vi "Apply Gradients.vi"(10 "Hardware Parameters In":T2={"Scan Calibration [G/V]"=0.0, "Modulation Calibration [G/V]"=0.0, "Modulation Phase [deg]"=0.0, "Modulation Frequency [Hz]"=0.0, "Attenuation [dB]"=0, "Input Channel Count"=0, "Time constant"=7, "Sensitivity"=17, "Frequency Output Voltage [V]"=0.0, "Phase Output Voltage [V]"=0.0, "Lock-in Offset Compensation"=FALSE, "RF [GHz]"=0.0, "Q Start"=0.0, "Q End"=0.0, "Balance"=0.0, "Phase Error"=0.0, "AFC Error"=0.0, "AFC"=FALSE, "Magnet Rotation"=FALSE, "Balance Scaling Factor"=1.0, "Phase Error Scaling Factor"=1.0, "AFC Error Scaling Factor"=1.0, "Frequency Counter ID"="", "Sweep Waveform"=enum."Sawtooth", "Q-Factor Scale"=0.0, " Q-Data Scale"=0.0, " Q-Data Offset"=0.0, "Magnet Rotation Slope"=0.0, "Magnet Rotation Offset"=0.0, "Phase Sweep Resolution"=0.0, "Hardware Version Number"="", "Spectrometer ID Number"=0, "Spectrometer Name"="", "Lock in Saturation"=0.0, "Balance Threshold"=0.0, "Phase Error Threshold"=0.0, "AFC Error Threshold"=0.0, "Linear Actuator Length"=0.0, "Lock-in OK?"=FALSE, "Ignore Lock-in Comm. Failure"=FALSE, "Gradient Addresses"=[], "Gradient Calibrations [G/A*mm]"=[], "Gradient Power Supplies"=[], "Lock-in Address"="", "Magnet Type"=enum."RRI", "Camera Names"=[], "Sweep Limit [Gauss]"=0.0, "Modulation Limit [Gauss]"=0.0, "Balance Threshold Exceeded?"=FALSE, "Phase Threshold Exceeded?"=FALSE, "AFC Threshold Exceeded?"=FALSE, "Consecutive Re-tune attempts"=0, "Reverse Sweep Slope [sec]"=0.0, "Reverse Sweep Offset [G]"=0.0, "AFC Field Correction [V/MHz]"=0.0, "Active Gradients (X Y Z)"=[], "SpO2 Calibration [SpO2/V]"=1.0, "Heart Rate Calibration [BPM/V]"=1.0, "Thermocouple Channel"=""} {"Sensitivity" items=["", "2 nV", "5 nV", "10 nV", "20 nV", "50 nV", "100 nV", "200 nV", "500 nV", "1 uV", "2 uV", "5 uV", "10 uV", "20 uV", "50 uV", "100 uV", "200 uV", "500 uV", "1 mV", "2 mV", "5 mV", "10 mV", "20 mV", "50 mV", "100 mV", "200 mV", "500 mV", "1 V"]; "Time constant" items=["10 us", "20 us", "40 us", "80 us", "160 us", "320 us", "640 us", "5 ms", "10 ms", "20 ms", "50 ms", "100 ms", "200 ms", "500 ms", "1 s", "2 s", "5 s", "10 s", "20 s", "50 s", "100 s", "200 s", "500 s", "1 ks", "2 ks", "5 ks", "10 ks", "20 ks", "50 ks", "100 ks"]}, 11 "Acquisition Parameters In":T1={"Magnet Angle [deg]"=0.0, "Magnet Angles [deg]"=[], "DeltaVpp [v]"=0.0, "SEM [v]"=0.0, "DeltaVpp Thresh [v]"=0.0, "SEM Thresh [v]"=0.0, "Adaptive Processing"=FALSE, "Acquire Q"=FALSE, "Acquire Photos"=FALSE, "Adaptive Tuning"=FALSE, "Automated Matching"=FALSE, "X-Gradient [G/mm]"=0.0, "Y-Gradient [G/mm]"=0.0, "Z-Gradient [G/mm]"=0.0, "Central Field [G]"=0.0, "Scan Width [G]"=0.0, "Mod. Amp. [G]"=0.0, "Scan Time [s]"=0.0, "Pre-Scan Delay [ms]"=0, "Measurement Timeout [s]"=0.0, "Electromagnet Main Field [G]"=0.0, "Locked Central Field [G]"=0.0, "Scans Excluded"=0, "Scans Completed"=0, "No. Scans/Set"=0, "No. Scans for SNR"=0, "Field Locked Frequency [GHz]"=0.0, "Auto Set-based Field Center"=FALSE, "Prompt for oxy acquisition updates"=FALSE, "Oxy QA Scan?"=FALSE, "Exclude Bad Data"=FALSE, "Optimizing RF Power"=FALSE, "Gradients on/off"=FALSE, "Running Script"=TRUE, "Opto-Coupler Current [A]"=0.0, "Continuous Sweeping"=FALSE, "Sweep Rise Time [sec]"=0, "Reverse Sweep Central Field [G]"=0.0, "Forward Sweep Central Field [G]"=0.0, "Sweep Calibrated"=FALSE, "Modulation Calibrated"=FALSE, "First CheckCal Scan?"=FALSE, "AFC Field Correction"=FALSE, "OxyQAInit Scan Width [G]"=0.0, "OxyQAInit Mod. Amp. [G]"=0.0, "Scans Completed/Session"=0, "Acquire SpO2"=FALSE, "Acquire Temperature"=FALSE, "Over Mod"=FALSE} {"OxyQAInit Mod. Amp. [G]" min=0.0; "OxyQAInit Scan Width [G]" min=0.0; "Mod. Amp. [G]" min=0.0; "Scan Width [G]" min=0.0; "Measurement Timeout [s]" min=0.0; "Scan Time [s]" min=0.0; "Z-Gradient [G/mm]" min=0.0; "Y-Gradient [G/mm]" min=0.0; "X-Gradient [G/mm]" min=0.0; "SEM Thresh [v]" min=0.0; "DeltaVpp Thresh [v]" min=0.0; "SEM [v]" min=0.0}) -> (0 "error out":errorcluster)   [LabVIEW 2016]
uses:
  Types/Hardware Parameters.ctl
  Types/Acquisition Parameters.ctl
panel:
  # "Gradients"
  # "Field"
  # "Scans and Sets"
  # "Timing"
  # "Adaptive Dosimetric \nData Processing"
  # "Bridge I/O"
  # "Magnet Rotation"
  # "Field Calibration"
  # "Lock In Amplifier"
  # "Spectrometer Information"
  # "DAQ Settings"
  # "Gradient Coils and Field"
  # "X"
  # "Y"
  # "Z"
  # "Q-Measurements"
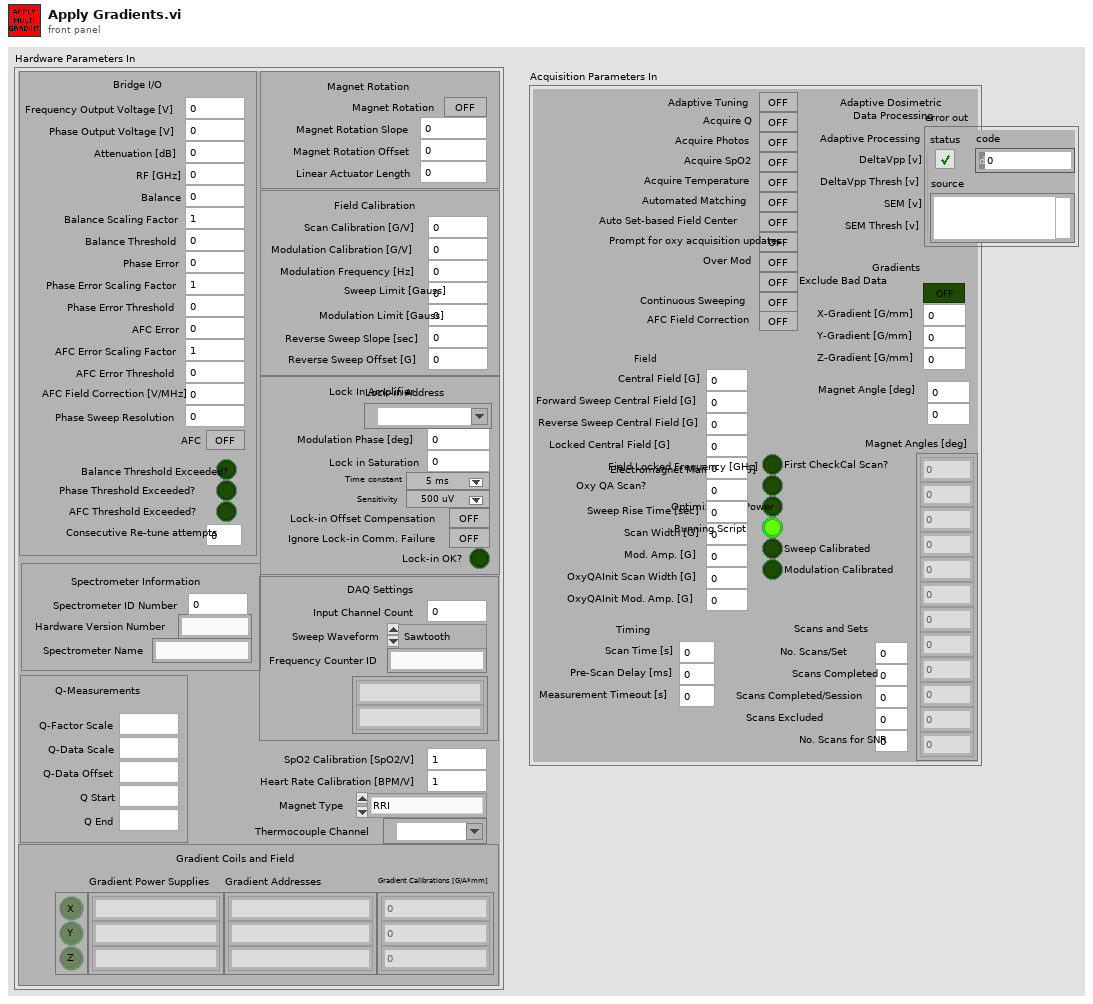
[diagram p1: front panel]
types:
  T1 = typedef "Acquisition Parameters.ctl" = cluster{"Magnet Angle [deg]":dbl, "Magnet Angles [deg]":dbl[], "DeltaVpp [v]":dbl, "SEM [v]":dbl, "DeltaVpp Thresh [v]":dbl, "SEM Thresh [v]":dbl, "Adaptive Processing":bool, "Acquire Q":bool, "Acquire Photos":bool, "Adaptive Tuning":bool, "Automated Matching":bool, "X-Gradient [G/mm]":dbl, "Y-Gradient [G/mm]":dbl, "Z-Gradient [G/mm]":dbl, "Central Field [G]":dbl, "Scan Width [G]":dbl, "Mod. Amp. [G]":dbl, "Scan Time [s]":dbl, "Pre-Scan Delay [ms]":u32, "Measurement Timeout [s]":dbl, "Electromagnet Main Field [G]":dbl, "Locked Central Field [G]":dbl, "Scans Excluded":u32, "Scans Completed":u32, "No. Scans/Set":u32, "No. Scans for SNR":u32, "Field Locked Frequency [GHz]":dbl, "Auto Set-based Field Center":bool, "Prompt for oxy acquisition updates":bool, "Oxy QA Scan?":bool, "Exclude Bad Data":bool, "Optimizing RF Power":bool, "Gradients on/off":bool, "Running Script":bool, "Opto-Coupler Current [A]":dbl, "Continuous Sweeping":bool, "Sweep Rise Time [sec]":u32, "Reverse Sweep Central Field [G]":dbl, "Forward Sweep Central Field [G]":dbl, "Sweep Calibrated":bool, "Modulation Calibrated":bool, "First CheckCal Scan?":bool, "AFC Field Correction":bool, "OxyQAInit Scan Width [G]":dbl, "OxyQAInit Mod. Amp. [G]":dbl, "Scans Completed/Session":u32, "Acquire SpO2":bool, "Acquire Temperature":bool, "Over Mod":bool}
  T2 = typedef "Hardware Parameters.ctl" = cluster{"Scan Calibration [G/V]":dbl, "Modulation Calibration [G/V]":dbl, "Modulation Phase [deg]":dbl, "Modulation Frequency [Hz]":dbl, "Attenuation [dB]":u16, "Input Channel Count":i32, "Time constant":u16, "Sensitivity":u16, "Frequency Output Voltage [V]":dbl, "Phase Output Voltage [V]":dbl, "Lock-in Offset Compensation":bool, "RF [GHz]":dbl, "Q Start":dbl, "Q End":dbl, "Balance":dbl, "Phase Error":dbl, "AFC Error":dbl, "AFC":bool, "Magnet Rotation":bool, "Balance Scaling Factor":dbl, "Phase Error Scaling Factor":dbl, "AFC Error Scaling Factor":dbl, "Frequency Counter ID":string, "Sweep Waveform":enum16{"Sine Wave", "Square Wave", "Sawtooth", "Triangle Wave"}, "Q-Factor Scale":dbl, " Q-Data Scale":dbl, " Q-Data Offset":dbl, "Magnet Rotation Slope":dbl, "Magnet Rotation Offset":dbl, "Phase Sweep Resolution":dbl, "Hardware Version Number":string, "Spectrometer ID Number":i32, "Spectrometer Name":string, "Lock in Saturation":dbl, "Balance Threshold":dbl, "Phase Error Threshold":dbl, "AFC Error Threshold":dbl, "Linear Actuator Length":dbl, "Lock-in OK?":bool, "Ignore Lock-in Comm. Failure":bool, "Gradient Addresses":string[], "Gradient Calibrations [G/A*mm]":dbl[], "Gradient Power Supplies":string[], "Lock-in Address":refnum<visa-resource-name>, "Magnet Type":enum16{"RRI", "BARDA", "Whole Body Permanent", "RRI Electromagnet"}, "Camera Names":string[], "Sweep Limit [Gauss]":dbl, "Modulation Limit [Gauss]":dbl, "Balance Threshold Exceeded?":bool, "Phase Threshold Exceeded?":bool, "AFC Threshold Exceeded?":bool, "Consecutive Re-tune attempts":i32, "Reverse Sweep Slope [sec]":dbl, "Reverse Sweep Offset [G]":dbl, "AFC Field Correction [V/MHz]":dbl, "Active Gradients (X Y Z)":bool[], "SpO2 Calibration [SpO2/V]":dbl, "Heart Rate Calibration [BPM/V]":dbl, "Thermocouple Channel":tag}
  T3 = enum16{"RRI", "BARDA", "Whole Body Permanent", "RRI Electromagnet"}
  T4 = enum16{"Main and Gradients", "Main Field", "Gradients"}
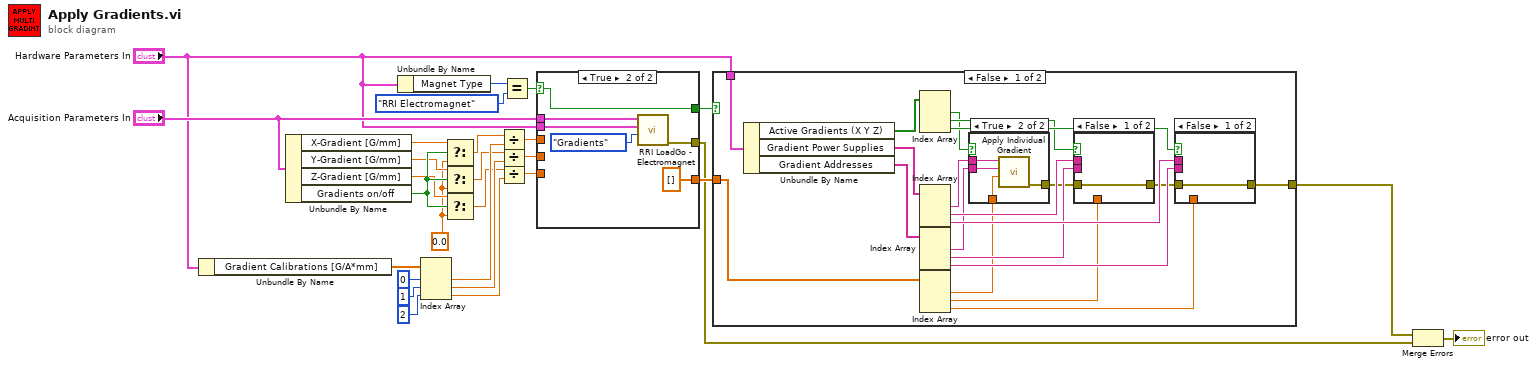
[diagram p0: block diagram]
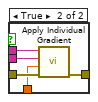
[diagram p2: hidden frame]
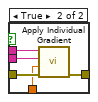
[diagram p3: hidden frame]
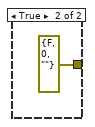
[diagram p5: hidden frame]
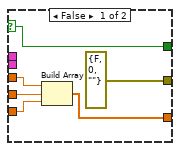
[diagram p6: hidden frame]
diagram:
  w1 = 0.0 ("t")
  n1 = Unbundle By Name("Hardware Parameters In") -> ("Gradient Calibrations [G/A*mm]"=w22:dbl[])
  n2 = Unbundle By Name("Acquisition Parameters In") -> ("X-Gradient [G/mm]"=w4:dbl, "Y-Gradient [G/mm]"=w3:dbl, "Z-Gradient [G/mm]"=w2:dbl, "Gradients on/off"=w8:bool)
  n3 = Unbundle By Name("Hardware Parameters In") -> ("Magnet Type"=w28:T3)
  n4 = Index Array(array=w22, index #1=0 ("index"), index #2=1 ("index"), index #3=2 ("index")) -> (element #1=w18:dbl, element #2=w17:dbl, element #3=w16:dbl)
  n5 = Select(t=w4, s=w8, f=w1) -> (s? t:f=w7:dbl)
  n6 = Select(t=w3, s=w8, f=w1) -> (s? t:f=w6:dbl)
  n7 = Select(t=w2, s=w8, f=w1) -> (s? t:f=w5:dbl)
  n8 = Divide(x=w7, y=w18) -> (x/y=w15:dbl)
  n9 = Divide(x=w6, y=w17) -> (x/y=w14:dbl)
  n10 = Divide(x=w5, y=w16) -> (x/y=w13:dbl)
  n11 = Equal?(x=w28, y=T3."RRI Electromagnet" ("Magnet Type")) -> (x = y?=w26:bool)
  n12 = case shown="True" w26 {
    selector: w26 -> [w33 w37]
    tunnel: "Acquisition Parameters In" -> [_ w35]
    tunnel: "Hardware Parameters In" -> [_ w39]
    tunnel: [errorcluster {"status"=FALSE, "code"=0, "source"=""} ("error out") w38] -> w10
    tunnel: [w33 w37] -> w25
    tunnel: w15 -> [w32 _]
    tunnel: w14 -> [w31 _]
    tunnel: w13 -> [w30 _]
    tunnel: [w29 dbl[] []] -> w12
    frame False {
      n13 = Build Array(w32, w31, w30) -> (w29:dbl[])
    }
    frame True {
      n14 = call "RRI LoadGo - Electromagnet.vi"("Control Coils"=T4."Gradients", "Hardware Parameters"=w39, "Acquisition Parameters"=w35) -> ("error out"=w38:errorcluster)  [unwired: 4 in]
    }
  }
  n15 = case shown="False" w25 {
    tunnel: [w48 errorcluster {"status"=FALSE, "code"=0, "source"=""} ("error out")] -> w11
    tunnel: "Hardware Parameters In" -> [w60 _]
    tunnel: w12 -> [w44 _]
    frame False {
      n16 = Unbundle By Name(w60) -> ("Active Gradients (X Y Z)"=w47:bool[], "Gradient Power Supplies"=w46:string[], "Gradient Addresses"=w45:string[])
      n17 = Index Array(array=w47) -> (element #1=w49:bool, element #2=w54:bool, element #3=w55:bool)  [unwired: 3 in]
      n18 = Index Array(array=w46) -> (element #1=w50:string, element #2=w58:string, element #3=w59:string)  [unwired: 3 in]
      n19 = Index Array(array=w45) -> (element #1=w51:string, element #2=w56:string, element #3=w57:string)  [unwired: 3 in]
      n20 = Index Array(array=w44) -> (element #1=w43:dbl, element #2=w42:dbl, element #3=w41:dbl)  [unwired: 3 in]
      n21 = case shown="True" w49 {
        tunnel: w50 -> [_ w76]
        tunnel: w51 -> [_ w75]
        tunnel: [_ w74] -> w52
        tunnel: w43 -> [_ w73]
        frame False {
        }
        frame True {
          n22 = call "Apply Individual Gradient.vi"("Current [A]"=w73, "Gradient Supply Address"=w75, "Gradient Supply Type"=w76) -> ("error out"=w74:errorcluster)  [unwired: 8 in]
        }
      }
      n23 = case shown="False" w54 {
        tunnel: w58 -> [_ w72]
        tunnel: w56 -> [_ w71]
        tunnel: [w67 w70] -> w53
        tunnel: w52 -> [w67 w69]
        tunnel: w42 -> [_ w68]
        frame False {
        }
        frame True {
          n24 = call "Apply Individual Gradient.vi"("error in"=w69, "Current [A]"=w68, "Gradient Supply Address"=w71, "Gradient Supply Type"=w72) -> ("error out"=w70:errorcluster)  [unwired: 7 in]
        }
      }
      n25 = case shown="False" w55 {
        tunnel: w59 -> [_ w66]
        tunnel: w57 -> [_ w65]
        tunnel: [w61 w64] -> w48
        tunnel: w53 -> [w61 w63]
        tunnel: w41 -> [_ w62]
        frame False {
        }
        frame True {
          n26 = call "Apply Individual Gradient.vi"("error in"=w63, "Current [A]"=w62, "Gradient Supply Address"=w65, "Gradient Supply Type"=w66) -> ("error out"=w64:errorcluster)  [unwired: 7 in]
        }
      }
    }
    frame True {
    }
  }
  n27 = Merge Errors(w11, w10) -> (→"error out":errorcluster)
